vi "Perform Action.vi"(8 "error in (no error)":errorcluster, 10 "Input":variant, 11 "Scope PXI Base CFG in":refnum<class "Scope PXI Base CFG.lvclass">) -> (0 "error out":errorcluster, 2 "Output":variant, 3 "Scope PXI Base CFG out":refnum<class "Scope PXI Base CFG.lvclass">)   [LabVIEW 2023, in "Scope PXI Base CFG.lvlib" / "Scope PXI Base CFG.lvclass"]
uses:
  Scope PXI Base CFG.lvclass
  Scope PXI Base CFG.lvclass/Scope PXI Base CFG.ctl
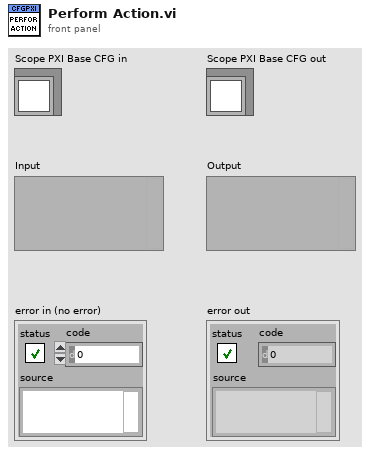
[diagram p1: front panel]
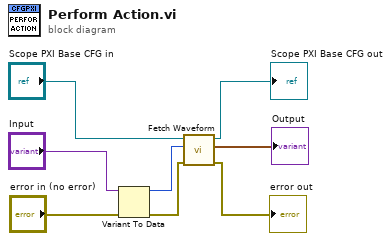
[diagram p0: block diagram]
diagram:
  n1 = Variant To Data(error in="error in (no error)", Variant="Input") -> (data=w4:u8, error out=w3:errorcluster)  [unwired: 1 in]
  n2 = call-dynamic "Fetch Waveform.vi"("error in (no error)"=w3, "Channel"=w4, "Scope PXI Base CFG in"="Scope PXI Base CFG in") -> ("error out"=→"error out":errorcluster, "Waveform"=→"Output":waveform(dbl), "Scope PXI Base CFG out"=→"Scope PXI Base CFG out":refnum<class "Scope PXI Base CFG.lvclass">)  [unwired: 6 in]
